vi "HMS_IPConfig.vi"(8 "error in (no error)":errorcluster) -> (0 "error out":errorcluster, 1 "PASS?":bool, 2 "standard output":string, 3 "standard error":string)   [LabVIEW 2016]
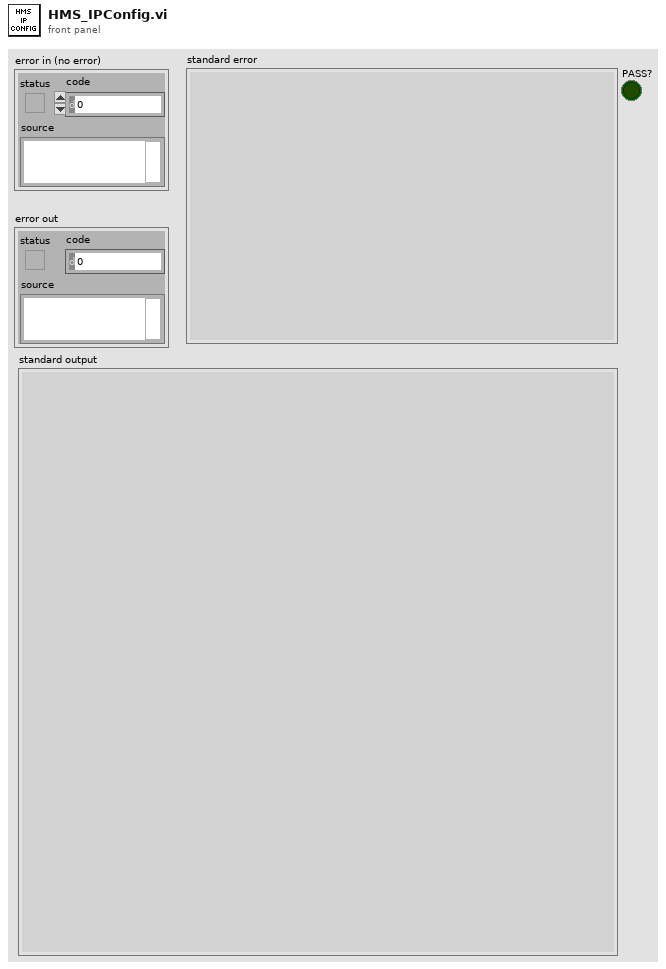
[diagram p1: front panel]
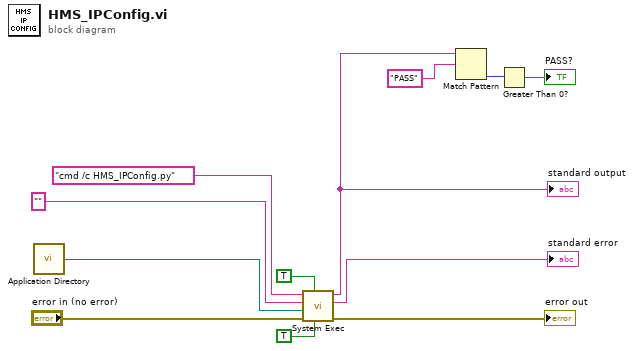
[diagram p0: block diagram]
diagram:
  n1 = call <vilib>:"Application Directory.vi"() -> ("Application Directory"=w1:path)
  n2 = call <vilib>:"System Exec.vi"("run minimized? (F)"=TRUE, "wait until completion? (T)"=TRUE ("run minimized? (F)"), "error in (no error)"="error in (no error)", "working directory"=w1, "standard input"="", "command line"="cmd /c HMS_IPConfig.py" ("name or relative path")) -> ("error out"=→"error out":errorcluster, "standard error"=→"standard error":string, "standard output"=w4:string)  [unwired: 2 in, 1 out]
  "standard output" <- w4
  n3 = Match Pattern(string=w4, regular expression="PASS") -> (offset past match=w3:i32)  [unwired: 1 in, 3 out]
  n4 = Greater Than 0?(x=w3) -> (x > 0?=→"PASS?":bool)
